vi "Actor Core.vi"(8 "error in":errorcluster, 11 "Viewer in":refnum<class "Viewer.lvclass">) -> (0 "error out":errorcluster={"status"=TRUE, "code"=1556, "source"="In Place Element Structure in Actor Framework.lvlib:Message Priority Queue.lvclass:Priority Dequeue.vi:2780005->Actor Framework.lvlib:Actor.lvclass:Actor Core.vi:5880001->UI Window.lvlib:UI Window.lvclass:Actor Core.vi:5880001->Viewer.lvlib:Viewer.lvclass:Actor Core.vi"}, 3 "Actor out":refnum<class "Actor.lvclass">)   [LabVIEW 2018, in "Viewer.lvlib" / "Viewer.lvclass"]
doc: "(<B>Filename</B>: Actor Framework.lvlib:Actor.lvclass:Actor Core.vi)\n\nReceives messages to the actor, reacts to them, and initiates any error handling that may shut the actor down.\n\nDescendant classes may override this VI to append parallel tasks for the actor to complete while it handles messages. Overrides use the Call Parent Method node."
uses:
  Viewer.lvclass
  C:/Program Files/National Instruments/LabVIEW 2018/vi.lib/ActorFramework/Actor/Actor.lvclass
  C:/LVFAST FLASH/Flash Gordon v0.6.1b/User Interface/UI Window/UI Window.lvclass
  <vilib>/ActorFramework/Actor/Actor.lvclass
  Resources/Type Defs/Color Map.ctl
  <vilib>/ActorFramework/Actor/Actor.lvclass/Actor.ctl
  Viewer.lvclass/Viewer.ctl
  <vilib>/ActorFramework/Message Enqueuer/Message Enqueuer.lvclass/Message Enqueuer.ctl
  <vilib>/ActorFramework/Message Enqueuer/Enqueue.vi
  Application Messages/Live Button Off Msg/Live Button Off Msg.lvclass
  C:/Program Files/National Instruments/LabVIEW 2018/vi.lib/ActorFramework/Message/Message.lvclass
  Application Messages/Stop Focus Indicator Msg/Stop Focus Indicator Msg.lvclass
  Application Messages/Start Focus Indicator Msg/Start Focus Indicator Msg.lvclass
  <vilib>/ActorFramework/Message Priority Queue/Priority Enqueue.vi
  Resources/GLOBAL/GLOBAL Time-critical.vi
  UI Window/UI Window.lvclass
panel:
  in  "Force Resize":bool
  out "x-y":u32
  in  "Stop Loop":bool
  in  "Reset View":bool
  in  "Autoscale":bool=TRUE
  in  "Range (bits)":T1(ring)=enum."13"
  in  "Color Map":T2=enum."Fire"
  in  "Stop?":bool=TRUE
  out "Histogram":T3(graph)
  out "Color Map":dbl[][](graph)
  in  "Focus":bool
  in  "Scaling":dbl=1.0
  in  "Channel 2":u16(ring) items=["Cy3"]
  in  "Channel 1":u16(ring) items=["Cy3"]
  in  "Alignment Mode":bool
  out "Intensity Graph":dbl[][](graph)
  # "|"
  # "-("
  # "x"
  # ")|"
  # "(Experimental)"
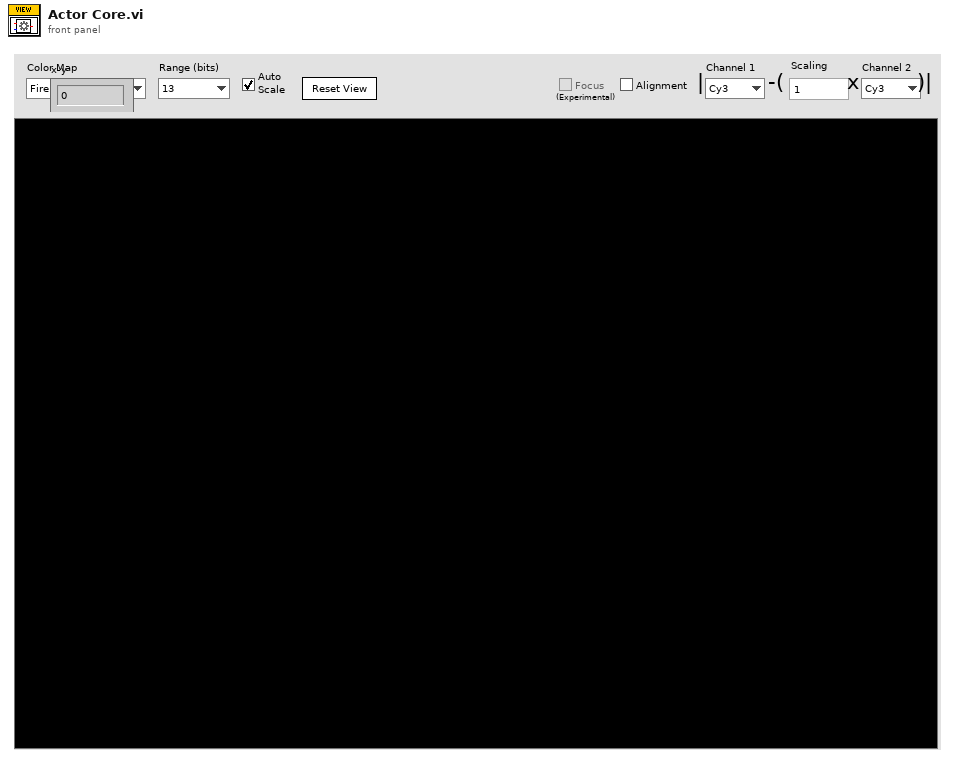
[diagram p1: front panel]
types:
  T1 = enum16{"16", "15", "14", "13", "12", "11", "10", "9", "8"}
  T2 = typedef "Color Map.ctl" = enum16{"Boring", "Fire", "Crazy", "Asylum", "Cubehelix", "Red", "Green", "Blue"}
  T3 = cluster{"X Values":dbl[], "Histogram: h(x)":i32[]}
  T4 = enum16{"None", "On Hover", "On Key Focus", "On Hover or Key Focus"}
  T5 = typedef "Physical Camera Assignment.ctl" = cluster{"Channel Name":string, "Camera Type":T6, "Serial Number":string, "Flip Vertically":bool, "Flip Horizontally":bool}
  T6 = typedef "Camera Type.ctl" = enum16{"Orca-Flash 4.0 V2"}
  T7 = typedef "eventvkey.ctl" = enum16{"ASCII", "Enter", "Return", "Shift", "Ctrl", "Alt", "Cmd", "Opt", "Caps", "NumLock", "Clear", "Break", "Up", "Down", "Left", "Right", "Insert", "Delete", "Home", "End", "PageUp", "PageDown", "Escape", "Help", "Pause", "ScrollLock", "F1", "F2", "F3", "F4", "F5", "F6", "F7", "F8", "F9", "F10", "F11", "F12", "F13", "F14", "F15", "F16", "F17", "F18", "F19", "F20", "F21", "F22", "F23", "F24", "Play", "VolumeUp", "VolumeDown", "Mute", "Two Byte Char"}
  T8 = typedef "LVRectTypeDef.ctl" = cluster{"Left":i16, "Top":i16, "Right":i16, "Bottom":i16}
  T9 = cluster{"Scale Min":dbl, "Cursor.Cursor Position:Cursor X":dbl}
  T10 = cluster{"Scale Max":dbl, "Cursor.Cursor Position:Cursor X":dbl}
  T11 = typedef "LVPoint32TypeDef.ctl" = cluster{"Horizontal":i32, "Vertical":i32}
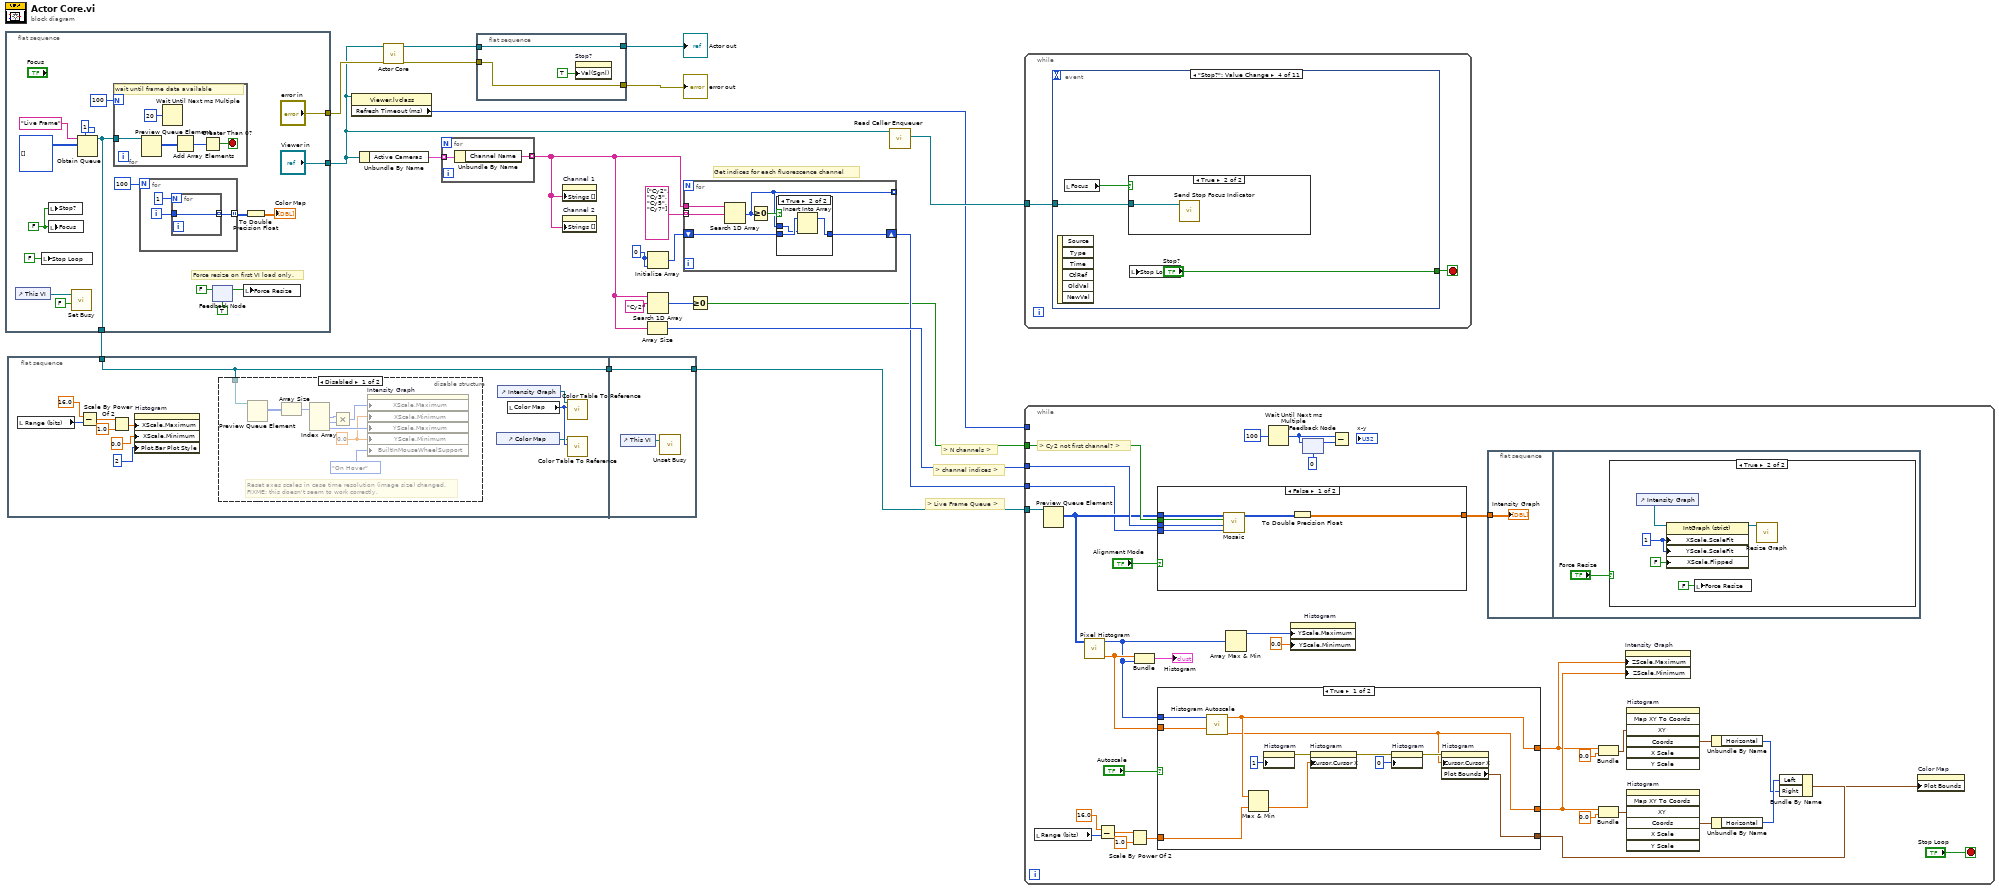
[diagram p0: block diagram]
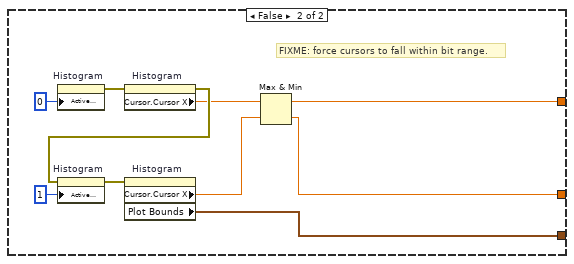
[diagram p5: hidden frame]
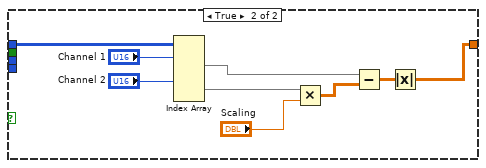
[diagram p6: hidden frame]
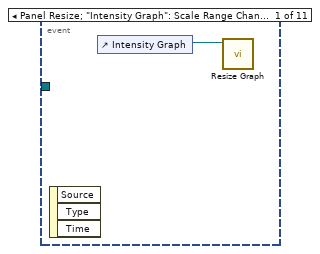
[diagram p7: hidden frame]
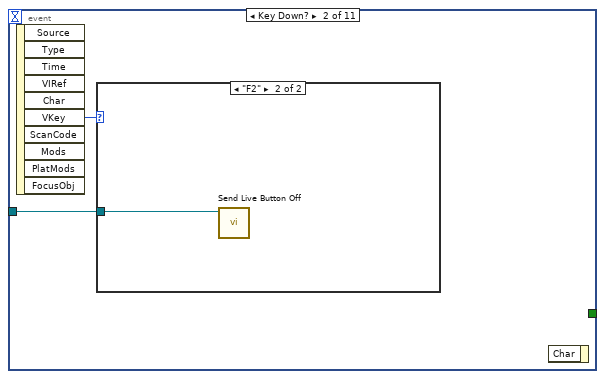
[diagram p8: hidden frame]
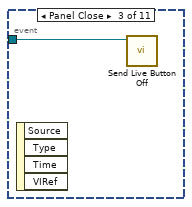
[diagram p10: hidden frame]
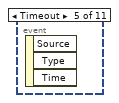
[diagram p12: hidden frame]
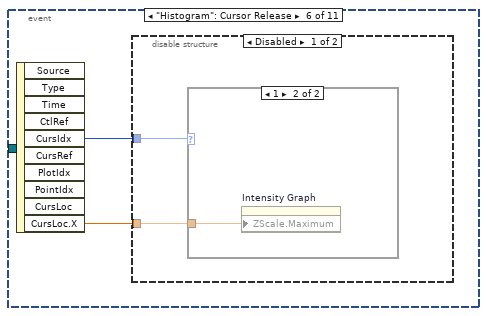
[diagram p13: hidden frame]
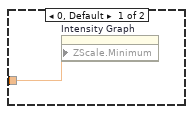
[diagram p14: hidden frame]
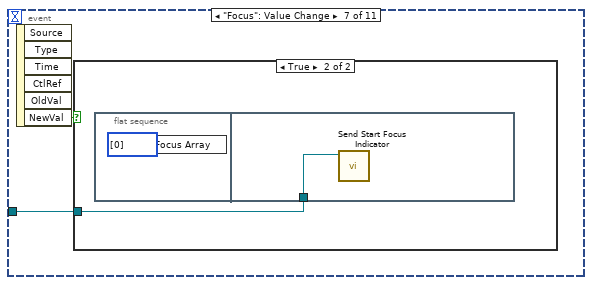
[diagram p16: hidden frame]
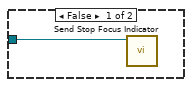
[diagram p17: hidden frame]
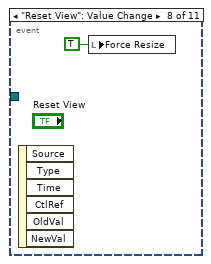
[diagram p18: hidden frame]
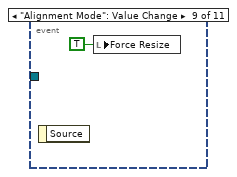
[diagram p19: hidden frame]
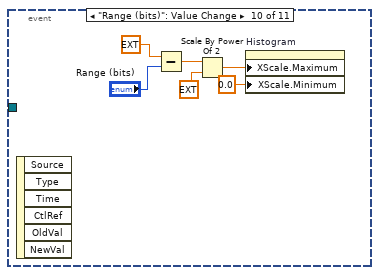
[diagram p20: hidden frame]
diagram:
  w13 = 0
  # "> N channels >"
  # "> channel indices >"
  # "Get indices for each fluorescence channel"
  # "> Live Frame Queue >"
  n1 = flat-sequence {
    tunnel: ["error in"] -> w21
    tunnel: ["Viewer in"] -> w5
    tunnel: [w28] -> w2
    frame #0 {
      w32 = FALSE ("Stop?")
      # "Force resize on first VI load only."
      n2 = control-ref of="This VI"() -> (w26:refnum<vi>)
      n3 = local write "Stop Loop"(FALSE ("Stop Loop")) -> ()
      n4 = local write "Stop?"(w32) -> ()
      n5 = local write "Focus"(w32) -> ()
      n6 = call <vilib>:"Set Busy.vi"("disable click? (T)"=FALSE, "VI reference (current VI)"=w26) -> ()  [unwired: 8 in, 2 out]
      n7 = Obtain Queue(max queue size (-1, unlimited)=1, name (unnamed)="Live Frame", element data type=u16[][][] [] ("element")) -> (queue out=w28:refnum<queue>)  [unwired: 2 in, 2 out]
      n8 = for {
        N: 100 -> [_]
        tunnel: w28 -> [w40]
        stop <- w39 stop-if-true
        # "wait until frame data available"
        n9 = Preview Queue Element(queue=w40) -> (element=w41:u16[][][])  [unwired: 2 in, 3 out]
        n10 = Wait Until Next ms Multiple(millisecond multiple=u32 20) -> ()  [unwired: 1 out]
        n11 = Add Array Elements(numeric array=w41) -> (sum=w43:u16)
        n12 = Greater Than 0?(x=w43) -> (x > 0?=w39:bool)
      }
      n13 = for {
        N: 100 -> [_]
        tunnel: [w45] -> w36 mode=indexing
        i -> [w46]
        n14 = for {
          N: 1 -> [_]
          tunnel: w46 -> [w47]
          tunnel: [w47] -> w45 mode=indexing
        }
      }
      n15 = feedback #1(TRUE) -> (w25:bool)
      n16 = feedback-in #1(FALSE) -> ()
      n17 = local write "Force Resize"(w25) -> ()
      n18 = To Double Precision Float(number=w36) -> (double precision float=→"Color Map":dbl[][])
    }
  }
  n19 = flat-sequence {
    tunnel: w2 -> [w49]
    tunnel: [w49] -> w1
    tunnel: [w69] -> w4
    tunnel: w1 -> [w69]
    frame #0 {
      n20 = local read "Range (bits)"() -> (w58:T1)
      n21 = Subtract(x=16.0, y=w58) -> (x-y=w56:dbl)
      n22 = Scale By Power Of 2(n=w56, x=1.0) -> (x*2^n=w57:dbl)
      n23 = property on="Histogram" class="XYGraph (strict)"("XScale.Maximum"=w57, "XScale.Minimum"=0.0 ("X Scale.Range:Minimum"), "Plot.Bar Plot Style"=u8 2) -> ()  [unwired: 2 in, 2 out]
      n24 = disable-structure shown="Disabled" {
        disable-tunnel: w49 -> [w67 _]
        frame Disabled {
          w60 = 0.0 ("X Scale.Range:Minimum")
          # "Reset axes scales in case time resolution (image size) changed.\nFIXME: this doesn't seem to work correctly."
          n25 = Preview Queue Element(queue=w67) -> (element=w66:u16[][][])  [unwired: 2 in, 3 out]
          n26 = Array Size(array=w66) -> (size(s)=w61:i32[])
          n27 = Index Array(array=w61) -> (element #1=w62:i32, element #2=w63:i32, element #3=w65:i32)  [unwired: 3 in]
          n28 = Multiply(x=w62, y=w63) -> (x*y=w64:i32)
          n29 = property on="Intensity Graph" class="IntGraph (strict)"("XScale.Maximum"=w64, "XScale.Minimum"=w60, "YScale.Maximum"=w65, "YScale.Minimum"=w60, "BuiltInMouseWheelSupport"=T4."On Hover" ("Built-In Mouse Wheel Support")) -> ()  [unwired: 2 in, 2 out]
        }
        frame Enabled {
        }
      }
      n30 = control-ref of="Color Map"() -> (w51:refnum<vi>)
      n31 = control-ref of="Intensity Graph"() -> (w50:refnum<vi>)
      n32 = local read "Color Map"() -> (w52:T2)
      n33 = call "Color Table To Reference.vi"("Color Map"=w52, "Intensity Graph Reference"=w50) -> ()  [unwired: 10 in]
      n34 = call "Color Table To Reference.vi"("Color Map"=w52, "Intensity Graph Reference"=w51) -> ()  [unwired: 10 in]
    }
    frame #1 {
      n35 = control-ref of="This VI"() -> (w68:refnum<vi>)
      n36 = call <vilib>:"Unset Busy.vi"("VI reference (current VI)"=w68) -> ()  [unwired: 10 in, 1 out]
    }
  }
  n37 = property class="Viewer.lvclass"(reference=w5) -> ("Refresh Timeout (ms)"=w6:i32)  [unwired: 1 in, 2 out]
  n38 = Unbundle By Name(w5) -> ("Active Cameras"=w15:T5[])
  n39 = call-parent "Actor Core.vi"("error in"=w21, "UI Window in"=w5) -> ("error out"=w19:errorcluster, "Actor out"=w20:refnum<class "Actor.lvclass">)  [unwired: 8 in]
  n40 = for {
    tunnel: w15 -> [w71] mode=indexing
    tunnel: [w70] -> w3 mode=indexing
    n41 = Unbundle By Name(w71) -> ("Channel Name"=w70:string)
  }
  n42 = flat-sequence {
    tunnel: w20 -> [w74]
    tunnel: w19 -> [w73]
    tunnel: [w74] -> w18
    tunnel: [w73] -> w17
    frame #0 {
      n43 = property on="Stop?" class="Bool (strict)"("Val(Sgnl)"=TRUE ("Stop?")) -> ()  [unwired: 2 in, 2 out]
    }
  }
  n44 = property on="Channel 1" class="Ring (strict)"("Strings []"=w3) -> ()  [unwired: 2 in, 2 out]
  n45 = property on="Channel 2" class="Ring (strict)"("Strings []"=w3) -> ()  [unwired: 2 in, 2 out]
  n46 = Array Size(array=w3) -> (size(s)=w9:i32)
  n47 = Initialize Array(w13, w13) -> (w12:i32[])
  n48 = Search 1D Array(1D array=w3, element="Cy2") -> (index of element=w10:i32)  [unwired: 1 in]
  n49 = for {
    tunnel: string[] ["Cy2", "Cy3", "Cy5", "Cy7"] -> [w79] mode=indexing
    tunnel: w3 -> [w80]
    shift-right: [w76] -> w8
    shift-left: w12 -> [w77]
    tunnel: [w75] -> _ mode=indexing
    n50 = Search 1D Array(1D array=w80, element=w79) -> (index of element=w75:i32)  [unwired: 1 in]
    n51 = Greater Or Equal To 0?(x=w75) -> (x >= 0?=w78:bool)
    n52 = case shown="True" w78 {
      tunnel: w77 -> [w81 w84]
      tunnel: w75 -> [_ w83]
      tunnel: [w81 w82] -> w76
      frame False {
      }
      frame True {
        n53 = Insert Into Array(array=w84, new element=w83) -> (w82:i32[])  [unwired: 1 in]
      }
    }
  }
  n54 = Greater Or Equal To 0?(x=w10) -> (x >= 0?=w7:bool)
  n55 = call <vilib>:"Read Caller Enqueuer.vi"("Actor"=w5) -> ("Caller Enqueuer"=w16:refnum<class "Message Enqueuer.lvclass">)  [unwired: 10 in]
  n56 = while {
    tunnel: w16 -> [w85]
    stop <- w86 stop-if-true
    n57 = event shown="[3] \"Stop?\": Value Change" {
      selector: _ -> [_ _ _ _ _ _ _ _ _ _ _]
      dyn-events: _ -> [_ _ _ _ _ _ _ _ _ _ _]
      timeout: _ -> [_ _ _ _ _ _ _ _ _ _ _]
      tunnel: [_ _ _ "Stop?" _ _ _ _ _ _ _] -> w86
      tunnel: w85 -> [_ w88 w91 w92 _ _ w102 _ _ _ _]
      event Panel Resize; "Intensity Graph": Scale Range Change {
        n58 = event-data() -> ()  [unwired: 1 in, 3 out]
        n59 = control-ref of="Intensity Graph"() -> (w87:refnum<vi>)
        n60 = call "Resize Graph.vi"("Intensity Graph Reference"=w87) -> ()  [unwired: 11 in]
      }
      event Key Down? {
        n61 = event-data() -> ("VKey"=w89:T7)  [unwired: 1 in, 9 out]
        n62 = case shown="\"F2\"" w89 {
          tunnel: w88 -> [_ w90]
          frame Default {
          }
          frame "F2" {
            n63 = call "Send Live Button Off.vi"("Message Enqueuer"=w90) -> ()  [unwired: 9 in, 2 out]
          }
        }
        n64 = event-data() -> ()  [unwired: 2 in, 1 out]
      }
      event Panel Close {
        n65 = event-data() -> ()  [unwired: 1 in, 4 out]
        n66 = call "Send Live Button Off.vi"("Message Enqueuer"=w91) -> ()  [unwired: 9 in, 2 out]
      }
      event "Stop?": Value Change {
        n67 = event-data() -> ()  [unwired: 1 in, 6 out]
        n68 = local read "Focus"() -> (w93:bool)
        n69 = case shown="True" w93 {
          tunnel: w92 -> [_ w95]
          frame False {
          }
          frame True {
            n70 = call "Send Stop Focus Indicator.vi"("Message Enqueuer"=w95) -> ()  [unwired: 9 in, 2 out]
          }
        }
        n71 = local write "Stop Loop"("Stop?") -> ()
      }
      event Timeout {
        n72 = event-data() -> ()  [unwired: 1 in, 3 out]
      }
      event "Histogram": Cursor Release {
        n73 = event-data() -> ("CursIdx"=w97:i32, "CursLoc.X"=w96:dbl)  [unwired: 1 in, 8 out]
        n74 = disable-structure shown="Disabled" {
          disable-tunnel: w97 -> [w99 _]
          disable-tunnel: w96 -> [w98 _]
          frame Disabled {
            n75 = case shown="1" w99 {
              tunnel: w98 -> [w100 w101]
              frame 0, Default {
                n76 = property on="Intensity Graph" class="IntGraph (strict)"("ZScale.Minimum"=w100) -> ()  [unwired: 2 in, 2 out]
              }
              frame 1 {
                n77 = property on="Intensity Graph" class="IntGraph (strict)"("ZScale.Maximum"=w101) -> ()  [unwired: 2 in, 2 out]
              }
            }
          }
          frame Enabled {
          }
        }
      }
      event "Focus": Value Change {
        n78 = event-data() -> ("NewVal"=w103:bool)  [unwired: 1 in, 5 out]
        n79 = case shown="True" w103 {
          tunnel: w102 -> [w104 w105]
          frame False {
            n80 = call "Send Stop Focus Indicator.vi"("Message Enqueuer"=w104) -> ()  [unwired: 9 in, 2 out]
          }
          frame True {
            n81 = flat-sequence {
              tunnel: w105 -> [w107]
              frame #0 {
                n82 = global write "GLOBAL Time-critical.vi" "Focus Array"(u16[] [0] ("Focus Array")) -> ()
              }
              frame #1 {
                n83 = call "Send Start Focus Indicator.vi"("Message Enqueuer"=w107) -> ()  [unwired: 9 in, 2 out]
              }
            }
          }
        }
      }
      event "Reset View": Value Change {
        n84 = event-data() -> ()  [unwired: 1 in, 6 out]
        n85 = local write "Force Resize"(TRUE ("Force Resize")) -> ()
      }
      event "Alignment Mode": Value Change {
        n86 = event-data() -> ()  [unwired: 1 in, 1 out]
        n87 = local write "Force Resize"(TRUE ("Force Resize")) -> ()
      }
      event "Range (bits)": Value Change {
        n88 = event-data() -> ()  [unwired: 1 in, 6 out]
        n89 = Subtract(x=ext 16.0, y="Range (bits)") -> (x-y=w112:ext)
        n90 = Scale By Power Of 2(n=w112, x=ext 1.0) -> (x*2^n=w114:ext)
        n91 = property on="Histogram" class="XYGraph (strict)"("XScale.Maximum"=w114, "XScale.Minimum"=0.0 ("X Scale.Range:Minimum")) -> ()  [unwired: 2 in, 2 out]
      }
      event Value Change {
        n92 = event-data() -> ()  [unwired: 1 in, 6 out]
        n93 = control-ref of="Intensity Graph"() -> (w118:refnum<vi>)
        n94 = control-ref of="Color Map"() -> (w117:refnum<vi>)
        n95 = call "Color Table To Reference.vi"("Color Map"="Color Map", "Intensity Graph Reference"=w117) -> ()  [unwired: 10 in]
        n96 = call "Color Table To Reference.vi"("Color Map"="Color Map", "Intensity Graph Reference"=w118) -> ()  [unwired: 10 in]
      }
    }
  }
  n97 = while {
    tunnel: w9 -> [w153]
    tunnel: w8 -> [w119]
    tunnel: w7 -> [w152]
    tunnel: w6 -> [_]
    tunnel: w4 -> [w149]
    stop <- "Stop Loop" stop-if-true
    # "> Cy2 not first channel? >"
    n98 = local read "Range (bits)"() -> (w140:T1)
    n99 = Preview Queue Element(queue=w149) -> (element=w120:u16[][][])  [unwired: 2 in, 3 out]
    n100 = call "Pixel Histogram.vi"("input"=w120) -> ("X Values"=w125:dbl[], "Histogram: h(x)"=w124:i32[])  [unwired: 9 in]
    n101 = Subtract(x=16.0, y=w140) -> (x-y=w141:dbl)
    n102 = Scale By Power Of 2(n=w141, x=1.0) -> (x*2^n=w138:dbl)
    n103 = Bundle("X Values"=w125, "Histogram: h(x)"=w124) -> (→"Histogram":T3)  [unwired: 1 in]
    n104 = case shown="False" "Alignment Mode" {
      tunnel: w120 -> [w185 w197]
      tunnel: w153 -> [w183 _]
      tunnel: w119 -> [w184 _]
      tunnel: w152 -> [w188 _]
      tunnel: [w187 w191] -> w121
      frame False {
        n105 = call "Mosaic.vi"("channel indices"=w184, "N channels"=w183, "Cy2 first?"=w188, "image array"=w185) -> ("element out"=w186:u16[][])  [unwired: 7 in]
        n106 = To Double Precision Float(number=w186) -> (double precision float=w187:dbl[][])
      }
      frame True {
        n107 = Index Array(array=w197, index (dim 0) #1="Channel 1", index (dim 0) #2="Channel 2") -> (element #1=w189:u16[][], element #2=w190:u16[][])  [unwired: 4 in]
        n108 = Multiply(x=w190, y="Scaling") -> (x*y=w193:dbl[][])
        n109 = Subtract(x=w189, y=w193) -> (x-y=w192:dbl[][])
        n110 = Absolute Value(x=w192) -> (abs(x)=w191:dbl[][])
      }
    }
    n111 = case shown="True" "Autoscale" {
      tunnel: [w162 w174] -> w136
      tunnel: [w161 w173] -> w137
      tunnel: [w167 w177] -> w139
      tunnel: w125 -> [w165 _]
      tunnel: w124 -> [w166 _]
      tunnel: w138 -> [w164 _]
      frame True {
        n112 = call "Histogram Autoscale.vi"("X Values"=w165, "Histogram: h(x)"=w166) -> ("Scale Max"=w161:dbl, "Scale Min"=w162:dbl)  [unwired: 6 in]
        n113 = Max & Min(x=w162, y=w164) -> (min(x,y)=w163:dbl)  [unwired: 1 out]
        n114 = property on="Histogram" class="XYGraph (strict)"("Active Cursor"=u32 1) -> (error out=w169:errorcluster)  [unwired: 2 in, 1 out]
        n115 = property on="Histogram" class="XYGraph (strict)"(error in=w169, "Cursor.Cursor X"=w163) -> (error out=w170:errorcluster)  [unwired: 1 in, 1 out]
        n116 = property on="Histogram" class="XYGraph (strict)"(error in=w170, "Active Cursor"=u32 0) -> (error out=w168:errorcluster)  [unwired: 1 in, 1 out]
        n117 = property on="Histogram" class="XYGraph (strict)"(error in=w168, "Cursor.Cursor X"=w161) -> ("Plot Bounds"=w167:T8)  [unwired: 1 in, 2 out]
      }
      frame False {
        # "FIXME: force cursors to fall within bit range."
        n118 = property on="Histogram" class="XYGraph (strict)"("Active Cursor"=u32 0) -> (error out=w179:errorcluster)  [unwired: 2 in, 1 out]
        n119 = property on="Histogram" class="XYGraph (strict)"(error in=w179) -> (error out=w180:errorcluster, "Cursor.Cursor X"=w176:dbl)  [unwired: 1 in, 1 out]
        n120 = property on="Histogram" class="XYGraph (strict)"(error in=w180, "Active Cursor"=u32 1) -> (error out=w178:errorcluster)  [unwired: 1 in, 1 out]
        n121 = property on="Histogram" class="XYGraph (strict)"(error in=w178) -> ("Cursor.Cursor X"=w175:dbl, "Plot Bounds"=w177:T8)  [unwired: 1 in, 2 out]
        n122 = Max & Min(x=w176, y=w175) -> (max(x,y)=w174:dbl, min(x,y)=w173:dbl)
      }
    }
    n123 = Array Max & Min(array=w124) -> (max value=w128:i32)  [unwired: 3 out]
    n124 = Wait Until Next ms Multiple(millisecond multiple=u32 100 ("milliseconds to wait")) -> (millisecond timer value=w122:u32)
    n125 = property on="Histogram" class="XYGraph (strict)"("YScale.Maximum"=w128, "YScale.Minimum"=0.0 ("Y Scale.Range:Minimum")) -> ()  [unwired: 2 in, 2 out]
    n126 = feedback-in #2(w122) -> ()
    n127 = feedback #2(u32 0 ("millisecond timer value")) -> (w148:u32)
    n128 = Subtract(x=w122, y=w148) -> ()  [unwired: 1 out]
    n129 = flat-sequence {
      tunnel: w121 -> [w154]
      frame #0 {
        "Intensity Graph" <- w154
      }
      frame #1 {
        n130 = case shown="True" "Force Resize" {
          frame False {
          }
          frame True {
            w160 = u8 1 ("X Scale.Scale Fit")
            n131 = control-ref of="Intensity Graph"() -> (w157:refnum<vi>)
            n132 = property class="IntGraph (strict)"(reference=w157, "XScale.ScaleFit"=w160, "YScale.ScaleFit"=w160, "XScale.Flipped"=FALSE ("X Scale.Flipped")) -> (reference out=w159:refnum<vi>)  [unwired: 1 in, 1 out]
            n133 = local write "Force Resize"(FALSE ("Force Resize")) -> ()
            n134 = call "Resize Graph.vi"("Intensity Graph Reference"=w159) -> ()  [unwired: 11 in]
          }
        }
      }
    }
    n135 = Bundle("Scale Min"=w136, "Cursor.Cursor Position:Cursor X"=0.0) -> (w129:T9)  [unwired: 1 in]
    n136 = Bundle("Scale Max"=w137, "Cursor.Cursor Position:Cursor X"=0.0) -> (w130:T10)  [unwired: 1 in]
    n137 = property on="Intensity Graph" class="IntGraph (strict)"("ZScale.Maximum"=w136, "ZScale.Minimum"=w137) -> ()  [unwired: 2 in, 2 out]
    n138 = invoke on="Histogram" class="XYGraph (strict)" method="Map XY To Coords"("XY"=w129) -> ("Coords"=w131:T11)  [unwired: 6 in, 6 out]
    n139 = invoke on="Histogram" class="XYGraph (strict)" method="Map XY To Coords"("XY"=w130) -> ("Coords"=w132:T11)  [unwired: 6 in, 6 out]
    n140 = Unbundle By Name(w131) -> ("Horizontal"=w134:i32)
    n141 = Unbundle By Name(w132) -> ("Horizontal"=w135:i32)
    n142 = Bundle By Name(cluster=w139, "Left"=w135, "Right"=w134) -> (w126:T8)
    n143 = property on="Color Map" class="IntGraph (strict)"("Plot Bounds"=w126) -> ()  [unwired: 2 in, 2 out]
  }
  "error out" <- w17
  "Actor out" <- w18
